vi "PH_DataViewer.constructor.vi"(0 "name":string, 2 "data in":string, 5 "error in(no error)":errorcluster) -> (14 "i ref out":refnum<vi>, 16 "data out":string, 19 "error out":errorcluster)   [LabVIEW 2014, in "PH_DataViewer.lvlib"]
doc: "This class is forseen to inspect shot data. Several of them can be saved in ASCI format.\n\nThis class is part of the PHELIX user layer.\n\nauthor: Stefan Götte, GSI\n\nLicense Agreement for this software:\n\nCopyright (C)\nGesellschaft für Schwerionenforschung, GSI\nPlanckstr. 1\n64291 Darmstadt\nGermany\n\nContact: D.Beck@gsi.de \n\nThis program is free software; you can redistribute it and/or modify it under the terms of the \nGNU General Public License as published by the Free Software Foundation; either version 2 of \nthe license, or (at your option) any later version.\n\nThis program is distributed in the hope that it will be useful, but WITHOUT ANY WARRANTY; \nwithout even the implied warranty of MERCHANTABILITY or FITNESS FOR A PARTICULAR PURPOSE. See the GNU General License for more details (http://www.gnu.org).\n\nGesellschaft für Schwerionenforschung, GSI\nPlanckstr. 1, 64291 Darmstadt, Germany\nFor all questions and ideas contact: M.Richter@gsi.de, H.Brand@gsi.de or D.Beck@gsi.de.\nLast update: 16-JUN-2004"
uses:
  PH_DataViewer.lvlib
  CS_Core/CSObj/CSObj.lvlib
  CS_Core/BaseGUI/BaseGUI.lvlib
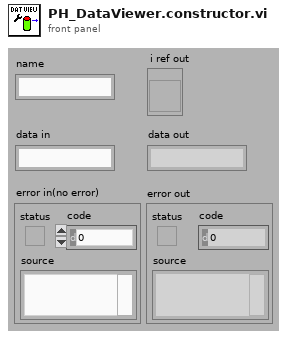
[diagram p1: front panel]
types:
  T1 = enum16{"SetAttribute", "GetAttribute", "CreateAttribute", "DestroyAttribute", "DestroyAllAtributes"}
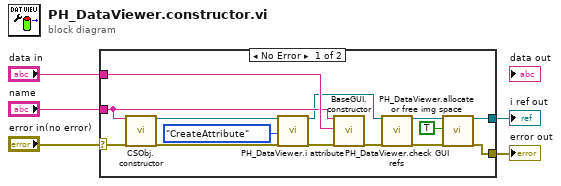
[diagram p0: block diagram]
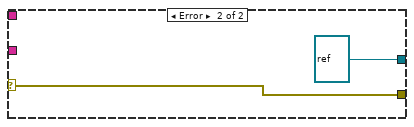
[diagram p2: hidden frame]
diagram:
  n1 = case shown="No Error" "error in(no error)" {
    selector: "error in(no error)" -> [w6 w21]
    tunnel: "data in" -> [w18 _]
    tunnel: "name" -> [w15 _]
    tunnel: [w13 w21] -> w3
    tunnel: [w12 refnum<vi> refnum ("i ref out")] -> w2
    frame No Error {
      n2 = call "CSObj.constructor.vi"("name"=w15, "error in (no error)"=w6) -> ("i ref out"=w17:refnum<vi>, "error out"=w16:errorcluster)  [unwired: 15 in, 1 out]
      n3 = call "PH_DataViewer.i attribute.vi"("VI Refnum"=w17, "Action"=T1."CreateAttribute", "error in (no error)"=w16) -> ("VI Refnum out"=w8:refnum<vi>, "error out"=w14:errorcluster)  [unwired: 14 in, 1 out]
      n4 = call "BaseGUI.constructor.vi"("name"=w15, "data in"=w18, "error in (no error)"=w14) -> ("error out"=w10:errorcluster)  [unwired: 14 in, 2 out]
      n5 = call "PH_DataViewer.check GUI refs.vi"("i ref in"=w8, "error in (no error)"=w10) -> ("i ref out"=w7:refnum<vi>, "error out"=w9:errorcluster)  [unwired: 16 in]
      n6 = call "PH_DataViewer.allocate or free img space.vi"("i ref in"=w7, "Allocate?"=TRUE, "error in (no error)"=w9) -> ("i ref out"=w12:refnum<vi>, "error out"=w13:errorcluster)  [unwired: 15 in]
    }
    frame Error {
    }
  }
  "i ref out" <- w2
  "error out" <- w3
